vi "报文测试.vi"() -> ()   [LabVIEW 2016, in "环境动力监测库.lvlib" / "NMEA.lvlib"]
uses:
  NMEA.lvlib
panel:
  out "接收数据区":string
  in  "关闭":bool
  in  "收方地址":string
  out "本机卡号":string
  in  "IC检测":bool
  in  "单次发送":bool
  in  "发送数据区":string
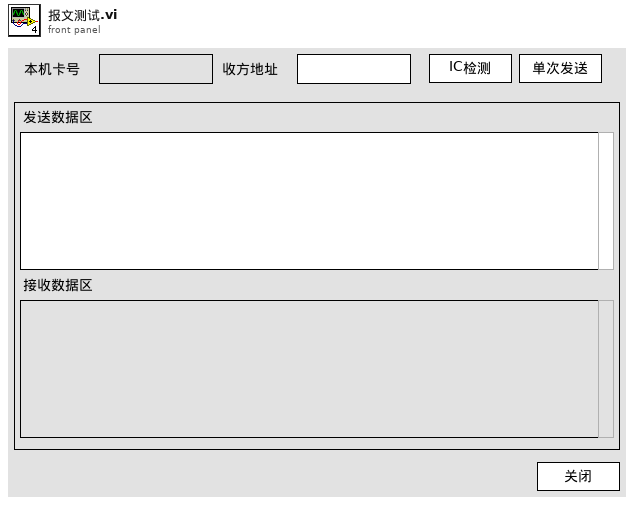
[diagram p1: front panel]
types:
  T1 = cluster{"指令":string, "长度":u16, "用户地址":string, "信息内容":cluster{"帧号":u8, "通播ID":u32, "用户特征":u8, "用户频度":u16, "通讯等级":u8, "加密标志":u8, "下属用户总数":u16}}
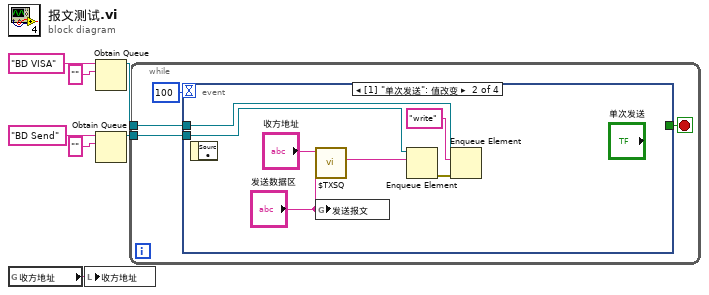
[diagram p0: block diagram]
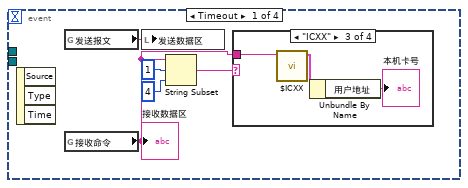
[diagram p2: hidden frame]
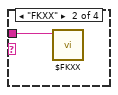
[diagram p4: hidden frame]
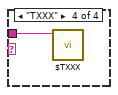
[diagram p5: hidden frame]
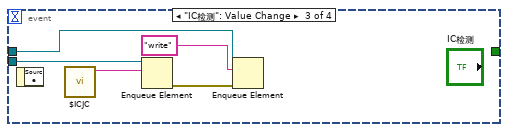
[diagram p6: hidden frame]
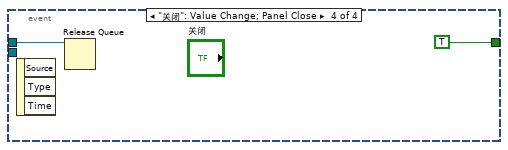
[diagram p7: hidden frame]
diagram:
  n1 = global read "断电保存全局变量.vi" "收方地址"() -> (w4:string)
  n2 = local write "收方地址"(w4) -> ()
  n3 = Obtain Queue(name (unnamed)="BD VISA" ("名称（未命名）"), element data type="" ("名称（未命名）")) -> (queue out=w5:refnum<queue>)  [unwired: 3 in, 2 out]
  n4 = Obtain Queue(name (unnamed)="BD Send" ("名称（未命名）"), element data type="" ("名称（未命名）")) -> (queue out=w1:refnum<queue>)  [unwired: 3 in, 2 out]
  n5 = while {
    tunnel: w5 -> [w9]
    tunnel: w1 -> [w8]
    stop <- w11 stop-if-true
    n6 = event shown="[1] \"单次发送\": 值改变" {
      selector: _ -> [_ _ _ _]
      dyn-events: _ -> [_ _ _ _]
      timeout: 100 -> [_ _ _ _]
      tunnel: [_ _ _ TRUE] -> w11
      tunnel: w9 -> [_ w27 w33 w34]
      tunnel: w8 -> [_ w25 w31 _]
      event Timeout {
        n7 = event-data() -> ()  [unwired: 1 in, 3 out]
        n8 = global read "发送报文全局变量.vi" "发送报文"() -> (w12:string)
        n9 = global read "发送报文全局变量.vi" "接收命令"() -> (w13:string)
        "接收数据区" <- w13
        n10 = local write "发送数据区"(w12) -> ()
        n11 = String Subset(string=w13, offset (0)=1 ("偏移量(0)"), length (rest)=4 ("长度（剩余）")) -> (substring=w15:string)
        n12 = case shown="\"ICXX\"" w15 {
          tunnel: w13 -> [_ w17 w18 w21]
          frame "假", Default {
          }
          frame "FKXX" {
            n13 = call "$FKXX.vi"("反馈信息"=w17) -> ()  [unwired: 10 in, 1 out]
          }
          frame "ICXX" {
            n14 = call "$ICXX.vi"("反馈信息"=w18) -> ("接收信息"=w20:T1)  [unwired: 10 in]
            n15 = Unbundle By Name(w20) -> ("用户地址"=→"本机卡号":string)
          }
          frame "TXXX" {
            n16 = call "$TXXX.vi"("反馈信息"=w21) -> ()  [unwired: 10 in, 1 out]
          }
        }
      }
      event "单次发送": Value Change {
        n17 = event-data() -> ()  [unwired: 1 in, 1 out]
        n18 = call "$TXSQ.vi"("电文内容"="发送数据区", "用户地址"="收方地址") -> ("字符串"=w24:string)  [unwired: 8 in, 1 out]
        n19 = global write "发送报文全局变量.vi" "发送报文"("发送数据区") -> ()
        n20 = Enqueue Element(queue=w25, element=w24) -> (error out=w23:errorcluster)  [unwired: 2 in, 2 out]
        n21 = Enqueue Element(queue=w27, element="write" ("元素"), error in (no error)=w23) -> ()  [unwired: 1 in, 3 out]
      }
      event "IC检测": Value Change {
        n22 = event-data() -> ()  [unwired: 1 in, 1 out]
        n23 = call "$ICJC.vi"() -> ("字符串"=w29:string)  [unwired: 11 in]
        n24 = Enqueue Element(queue=w31, element=w29) -> (error out=w30:errorcluster)  [unwired: 2 in, 2 out]
        n25 = Enqueue Element(queue=w33, element="write" ("元素"), error in (no error)=w30) -> ()  [unwired: 1 in, 3 out]
      }
      event "关闭": Value Change; Panel Close {
        n26 = event-data() -> ()  [unwired: 1 in, 3 out]
        n27 = Release Queue(queue=w34) -> ()  [unwired: 2 in, 3 out]
      }
    }
  }
